vi "Current control.vi"() -> ()   [LabVIEW 2019]
uses:
  <vilib>/rvi/Analysis/control/PID/Typedef/niFpgaPID_PIGains.ctl
  <vilib>/rvi/Analysis/control/PID/Typedef/niFpgaPID_OutputRange.ctl
  <vilib>/rvi/Emulation/niFpgaGetClockAttributes.vi
  <vilib>/rvi/Emulation/niFpgaSctlEmulationGetInTimedLoop.vi
  <vilib>/rvi/Emulation/niFpgaEmulationReportErrorSimple.vi
  <vilib>/rvi/eio/common/nirviEmuTemplateMethod_errors.vi
  <vilib>/rvi/Analysis/control/PID/SubVIs/niFpgaPID_PIWrapper.vi
  <vilib>/rvi/Emulation/niFpgaCriticalErrorInLSC.vi
  <vilib>/eio/EIONode/EIONode.xnode
panel:
  out "Direction":bool
  out "dutycycle":sgl(graph)
  out "error":sgl(graph)
  out "PID":sgl(graph)
  in  "output range":T1={"output high (Inf)"=inf, "output low (-Inf)"=-inf}
  out "Raw curent":sgl(graph)
  in  "current setpoint":sgl
  out "Raw voltage data":sgl(graph)
  out "filtered currrent":sgl(graph)
  out "setpoint":sgl(graph)
  in  "gains":T2 {"proportional gain" step=0.125}
  in  "measurement error":sgl
  in  "Process noise":sgl
  in  "off time":sgl
  in  "on time":sgl
  in  "stop":bool
  in  "PWM frequency":sgl
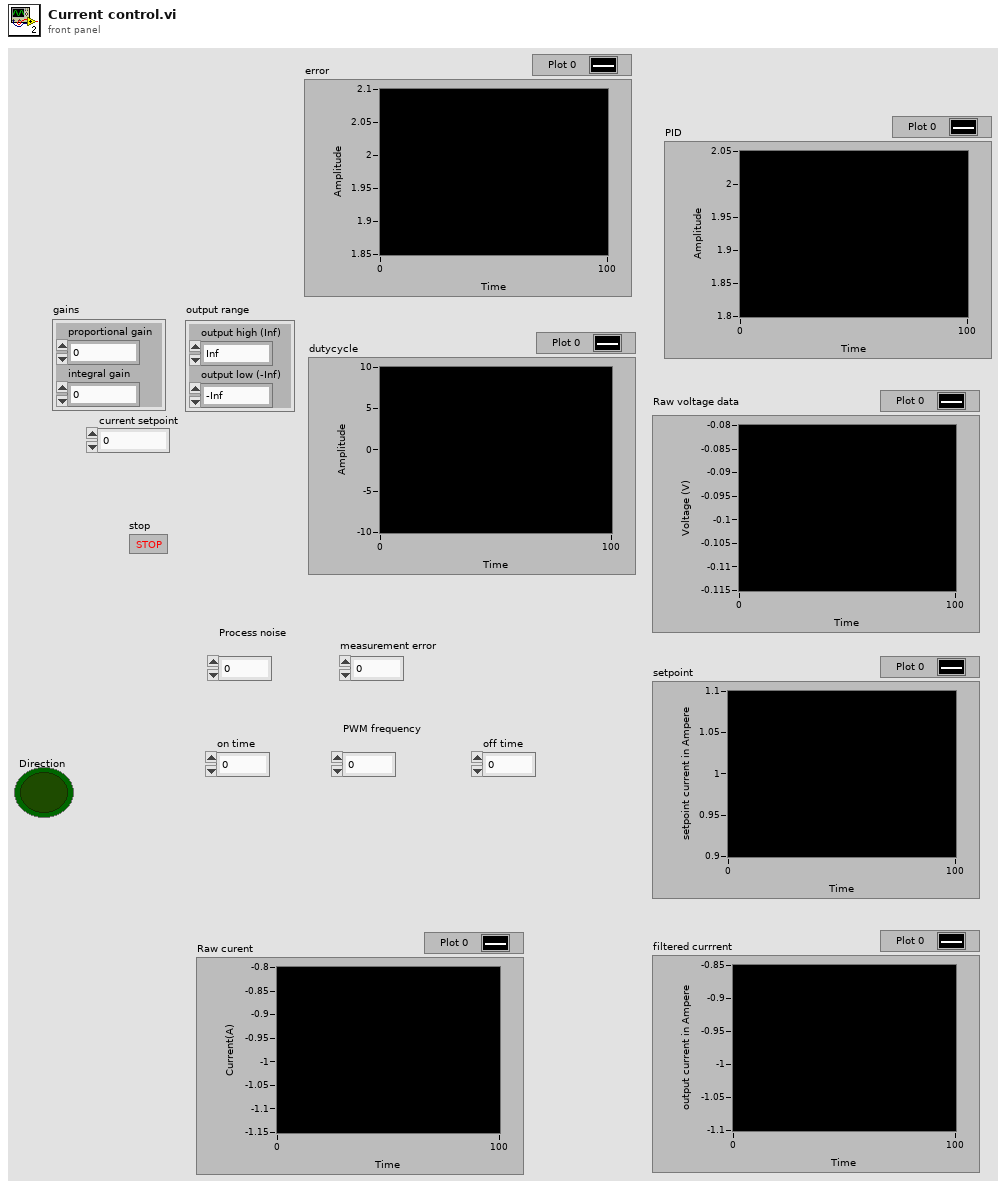
[diagram p1: front panel]
types:
  T1 = typedef "niFpgaPID_OutputRange.ctl" = cluster{"output high (Inf)":sgl, "output low (-Inf)":sgl}
  T2 = typedef "niFpgaPID_PIGains.ctl" = cluster{"proportional gain":sgl, "integral gain":sgl}
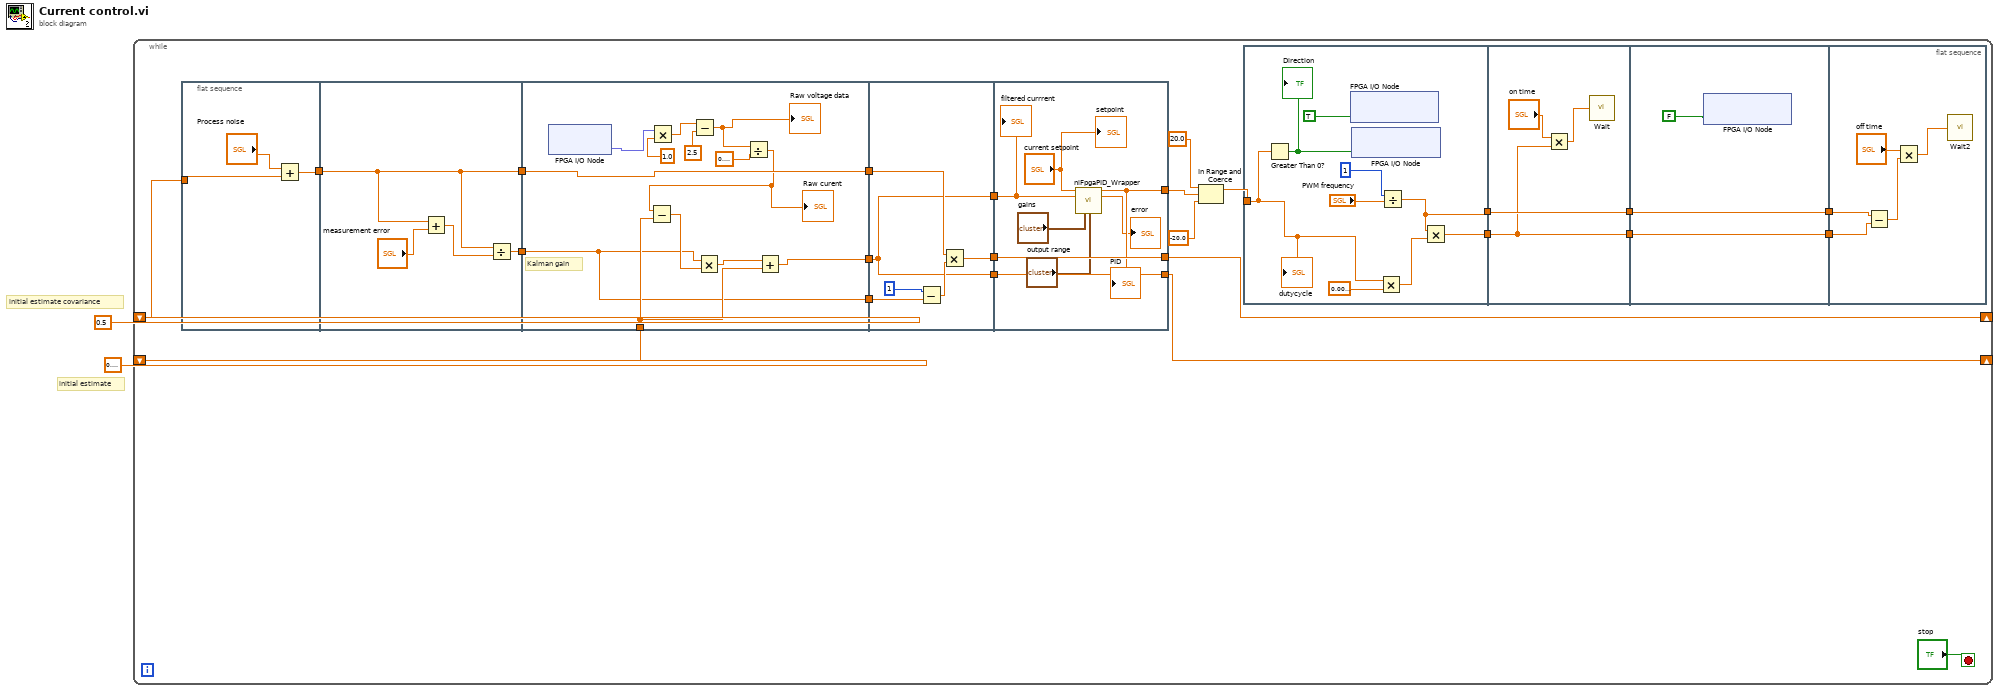
[diagram p0: block diagram]
diagram:
  # "initial estimate"
  # "initial estimate covariance"
  n1 = while {
    shift-right: [w4] -> _
    shift-left: sgl 0.1 -> [w15]
    shift-right: [w3] -> _
    shift-left: sgl 0.5 -> [w19]
    stop <- "stop" stop-if-true
    n2 = flat-sequence {
      tunnel: w19 -> [w28]
      tunnel: [w27] -> w18
      tunnel: w18 -> [w31]
      tunnel: [w31] -> w17
      tunnel: [w30] -> w16
      tunnel: w17 -> [w46]
      tunnel: w16 -> [w41]
      tunnel: w15 -> [w44]
      tunnel: [w46] -> w14
      tunnel: [w42] -> w13
      tunnel: [w41] -> w12
      tunnel: w14 -> [w49]
      tunnel: w13 -> [w47]
      tunnel: w12 -> [w52]
      tunnel: [w48] -> w11
      tunnel: [w47] -> w10
      tunnel: [w47] -> w9
      tunnel: [w59] -> w4
      tunnel: [w60] -> w3
      tunnel: w11 -> [w60]
      tunnel: w10 -> [w59]
      tunnel: w9 -> [w58]
      tunnel: [w56] -> w8
      frame #0 {
        n3 = Add(x="Process noise", y=w28) -> (x+y=w27:sgl)
      }
      frame #1 {
        n4 = Add(x=w31, y="measurement error") -> (x+y=w32:sgl)
        n5 = Divide(x=w31, y=w32) -> (x/y=w30:sgl)
      }
      frame #2 {
        # "Kalman gain"
        n6 = xnode "FPGA I/O Node"() -> ("AI0"=w37:fxp<+/-,24,5>)  [unwired: 1 in, 1 out]
        n7 = Multiply(x=w37, y=sgl 1.0) -> (x*y=w39:sgl)
        n8 = Subtract(x=w39, y=sgl 2.5) -> (x-y=w36:sgl)
        "Raw voltage data" <- w36
        n9 = Divide(x=w36, y=sgl 0.1) -> (x/y=w34:sgl)
        "Raw curent" <- w34
        n10 = Subtract(x=w34, y=w44) -> (x-y=w45:sgl)
        n11 = Multiply(x=w41, y=w45) -> (x*y=w43:sgl)
        n12 = Add(x=w43, y=w44) -> (x+y=w42:sgl)
      }
      frame #3 {
        n13 = Subtract(x=i16 1, y=w52) -> (x-y=w50:sgl)
        n14 = Multiply(x=w49, y=w50) -> (x*y=w48:sgl)
      }
      frame #4 {
        n15 = call-poly <vilib>:"niFpgaPID_Wrapper.vi"("setpoint"="current setpoint", "process variable"=w58, "gains"="gains", "output range"="output range") -> ("output"=w56:sgl, "error"=→"error":sgl)  [unwired: 9 in, 1 out]
        "PID" <- w56
        "setpoint" <- "current setpoint"
        "filtered currrent" <- w58
      }
    }
    n16 = In Range and Coerce(upper limit=sgl 20.0, x=w8, lower limit=sgl -20.0) -> (coerced(x)=w5:sgl)  [unwired: 1 out]
    n17 = flat-sequence {
      tunnel: [w65] -> w26
      tunnel: [w64] -> w25
      tunnel: w5 -> [w62]
      tunnel: w26 -> [w72]
      tunnel: w25 -> [w73]
      tunnel: [w72] -> w24
      tunnel: [w73] -> w23
      tunnel: w24 -> [w76]
      tunnel: w23 -> [w75]
      tunnel: [w76] -> w22
      tunnel: [w75] -> w21
      tunnel: w22 -> [w80]
      tunnel: w21 -> [w81]
      frame #0 {
        n18 = Greater Than 0?(x=w62) -> (x > 0?=w61:bool)
        "Direction" <- w61
        n19 = xnode "FPGA I/O Node"("RMC/DIO48"=TRUE) -> ()  [unwired: 1 in, 1 out]
        n20 = xnode "FPGA I/O Node"("RMC/DIO51"=w61) -> ()  [unwired: 1 in, 1 out]
        n21 = Multiply(x=w62, y=sgl 0.01) -> (x*y=w66:sgl)
        n22 = Divide(x=i16 1, y="PWM frequency") -> (x/y=w64:sgl)
        n23 = Multiply(x=w64, y=w66) -> (x*y=w65:sgl)
        "dutycycle" <- w62
      }
      frame #1 {
        n24 = Multiply(x="on time", y=w72) -> (x*y=w71:sgl)
        n25 = call "Wait"("Count(uSec)"=w71) -> ()  [unwired: 1 out]
      }
      frame #2 {
        n26 = xnode "FPGA I/O Node"("RMC/DIO48"=FALSE) -> ()  [unwired: 1 in, 1 out]
      }
      frame #3 {
        n27 = Subtract(x=w81, y=w80) -> (x-y=w79:sgl)
        n28 = Multiply(x="off time", y=w79) -> (x*y=w78:sgl)
        n29 = call "Wait2"("Count(uSec)"=w78) -> ()  [unwired: 1 out]
      }
    }
  }
